vi "EventDisplayWindow.vi"(8 "error in (no error)":errorcluster, 11 "Path to detector WRL file":path) -> (0 "error out":errorcluster)   [LabVIEW 2016]
uses:
  Typedefs/Coincidence.ctl
panel:
  in  "Events/sec":dbl=1.0
  in  "Firing color":u32(colorbox)=9809083
  in  "Idle color":u32(colorbox)=9809083
  in  "Enable Events":bool=TRUE
  in  "Scale":sgl=0.01
  out "Event display":refnum<vi>(3d-picture)
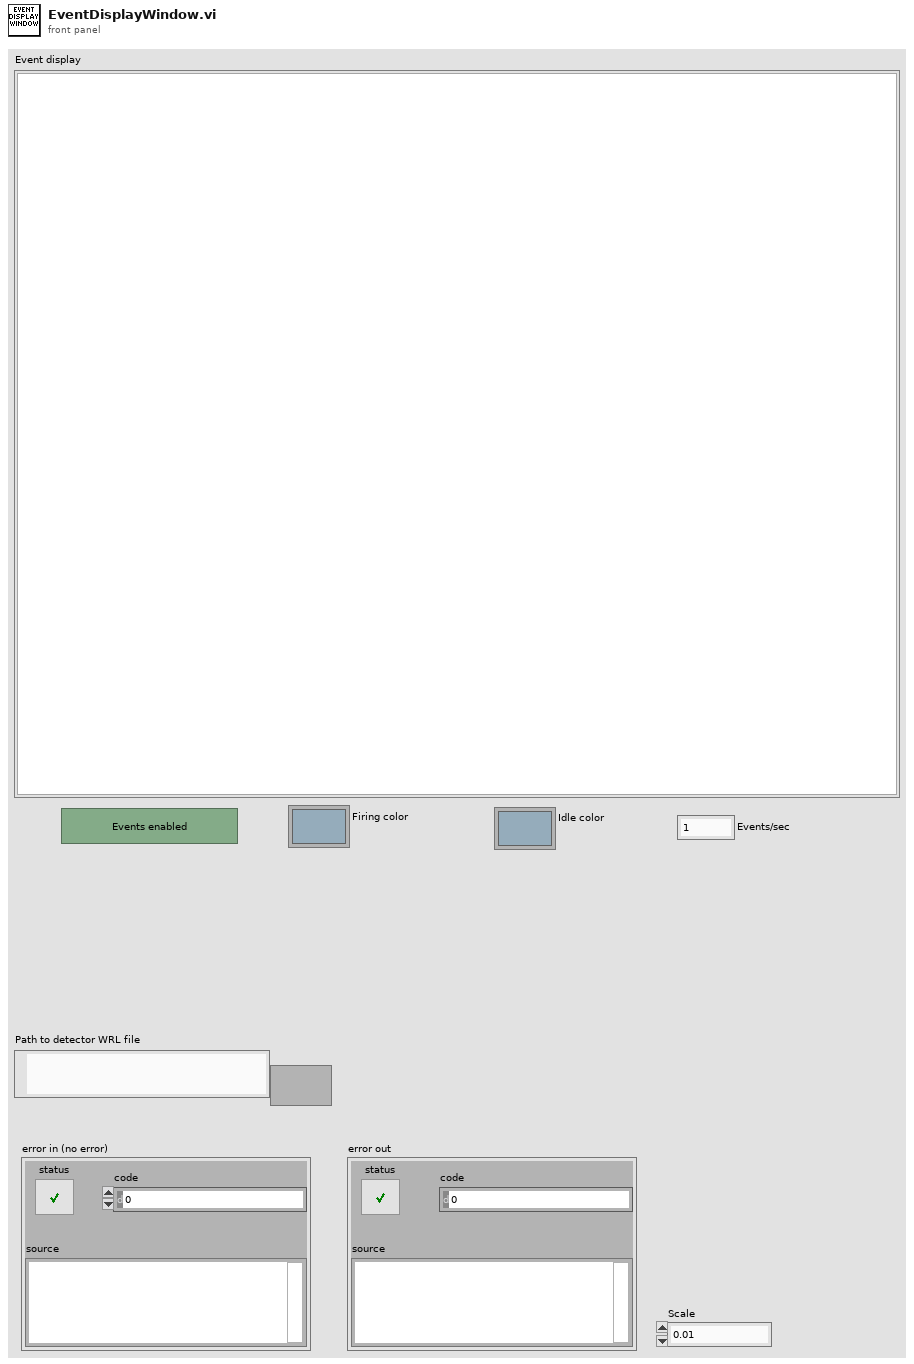
[diagram p1: front panel]
types:
  T1 = typedef "Coincidence.ctl" = cluster{"Primary ID":i8, "Muon hit time":u64, "Secondary ID":i8, "DeltaT":i32}
  T2 = cluster{"Simultaneus muon tracks":cluster{"Top coinc":T1, "Bottom coinc":T1}[]}[]
  T3 = cluster{"Frame color":u32, "Connectors color":u32, "Supports color":u32, "Bolts color":u32, "Scintillators color":u32, "Scintillator alpha":sgl}
  T4 = cluster{"Simultaneus muon tracks":cluster{"Top coinc":T1, "Bottom coinc":T1}[]}
  T5 = typedef "LVRGBAColorTypeDef.ctl" = cluster{"Red":sgl, "Green":sgl, "Blue":sgl, "Alpha":sgl}
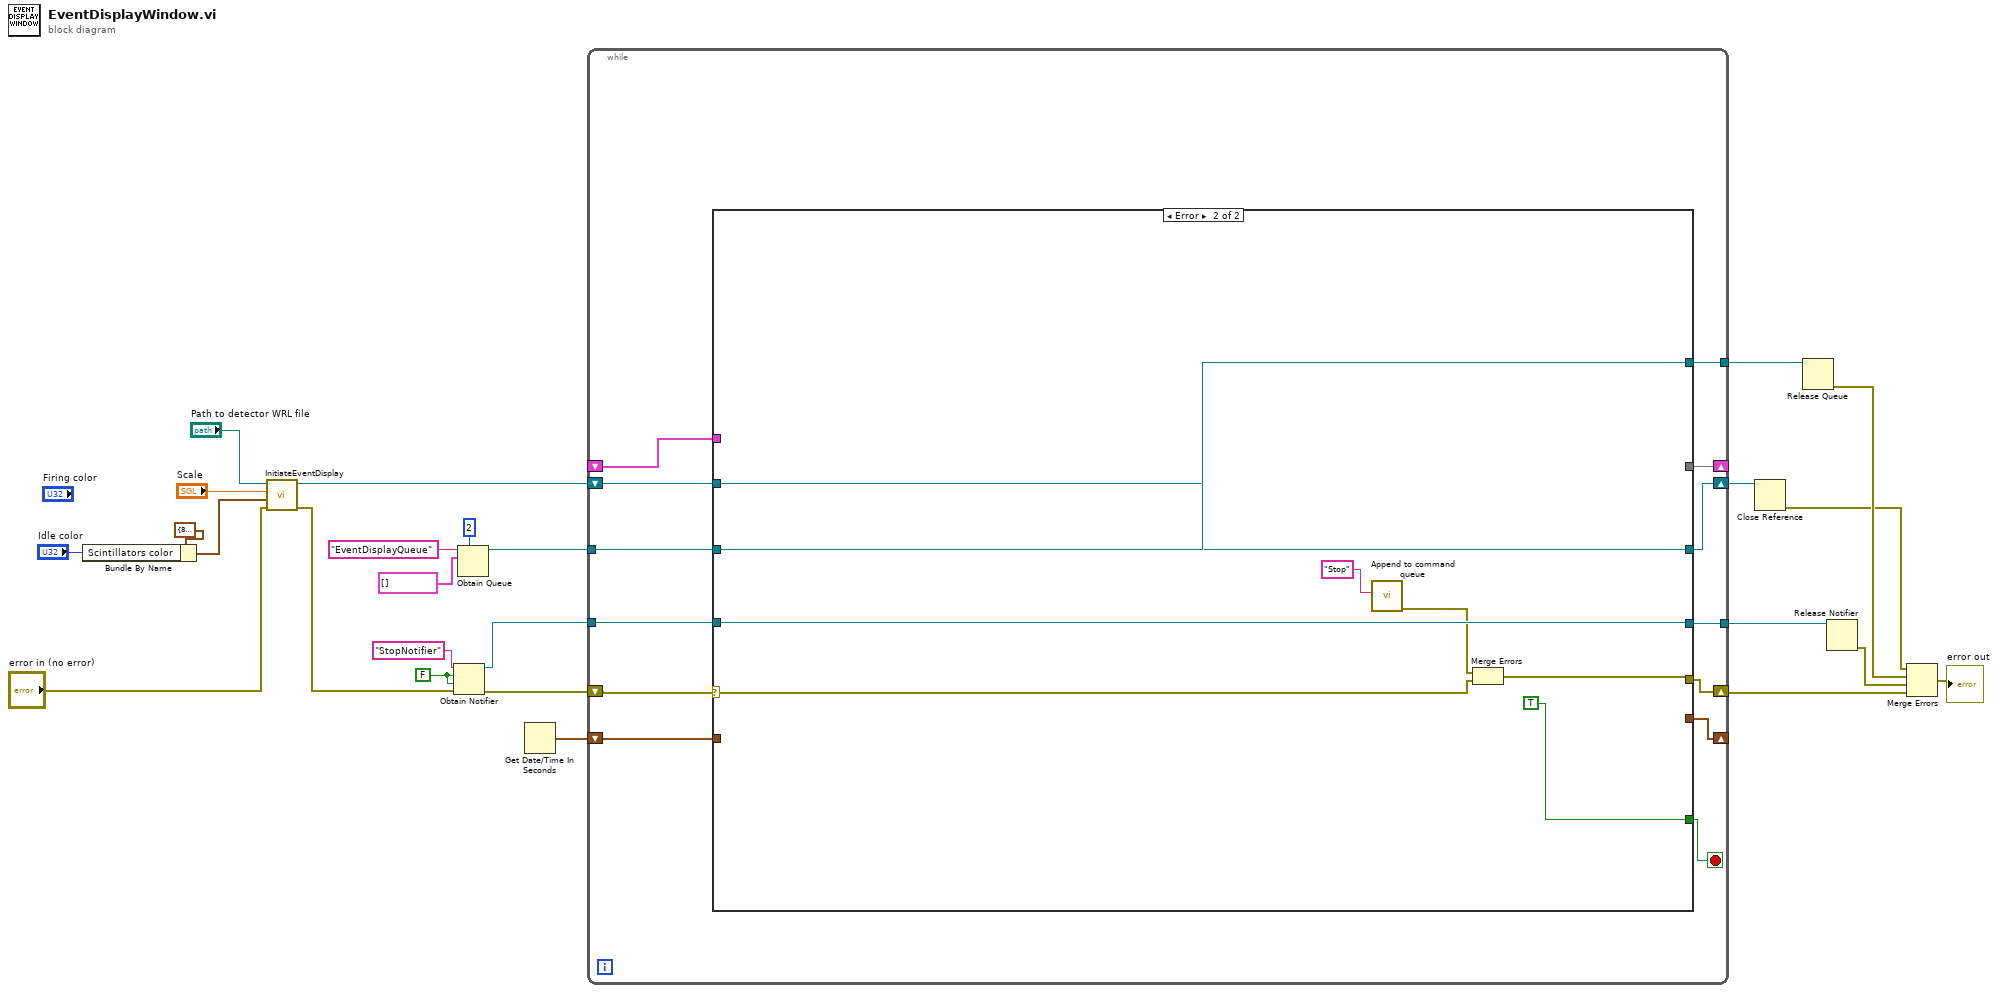
[diagram p0: block diagram]
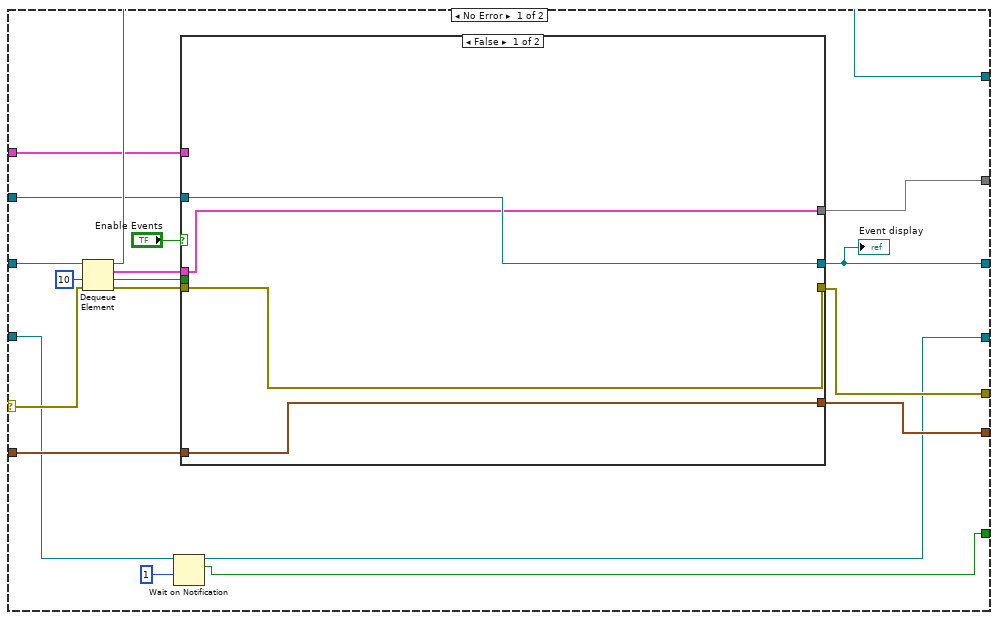
[diagram p2: hidden frame]
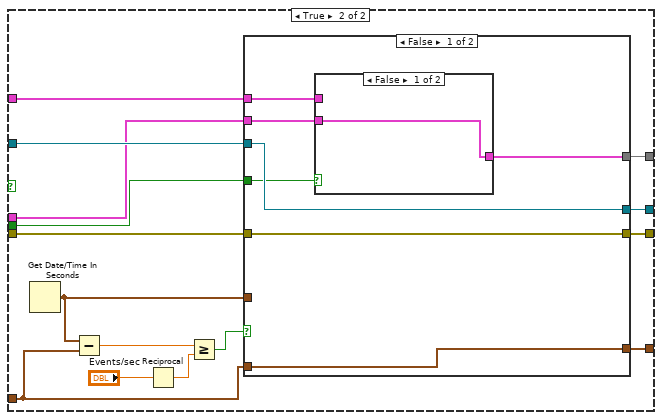
[diagram p3: hidden frame]
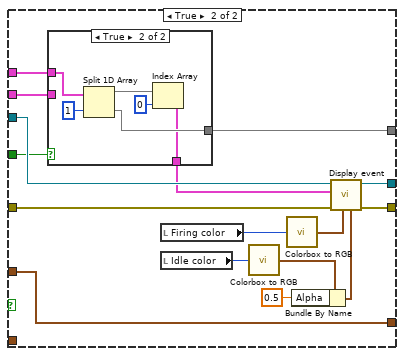
[diagram p5: hidden frame]
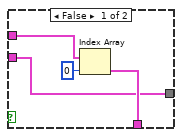
[diagram p6: hidden frame]
diagram:
  w24 = FALSE
  n1 = Bundle By Name(cluster=T3 {"Frame color"=8950380, "Connectors color"=5921370, "Supports color"=10395294, "Bolts color"=13487565, "Scintillators color"=9809083, "Scintillator alpha"=0.5} ("colors"), "Scintillators color"="Idle color") -> (w4:T3)
  n2 = call "InitiateEventDisplay.vi"("error in"="error in (no error)", "colors"=w4, "Scale"="Scale", "Path to detector WRL file"="Path to detector WRL file") -> ("error out"=w9:errorcluster, "Event Display Scene"=w8:refnum<vi>)  [unwired: 4 in]
  n3 = Obtain Notifier(name (unnamed)="StopNotifier", notification data type=w24, create if not found? (T)=w24, error in (no error)=w9) -> (notifier out=w22:refnum<notifier>, error out=w23:errorcluster)  [unwired: 1 out]
  n4 = Obtain Queue(max queue size (-1, unlimited)=2, name (unnamed)="EventDisplayQueue", element data type=T2 []) -> (queue out=w19:refnum<queue>)  [unwired: 2 in, 2 out]
  n5 = Get Date/Time In Seconds() -> (seconds since 1Jan1904=w2:timestamp)
  n6 = while {
    tunnel: w22 -> [w34]
    tunnel: w19 -> [w36]
    shift-right: [w35] -> w14
    shift-left: w23 -> [w38]
    tunnel: [w33] -> w17
    tunnel: [w32] -> w18
    shift-right: [w30] -> w7
    shift-left: w8 -> [w31]
    shift-right: [w28] -> _
    shift-left: w2 -> [w29]
    shift-right: [w26] -> _
    shift-left: _ -> [w27]
    stop <- w37 stop-if-true
    n7 = case shown="Error" w38 {
      selector: w38 -> [w55 w114]
      tunnel: [w44 TRUE] -> w37
      tunnel: w36 -> [w57 w113]
      tunnel: [w54 w116] -> w35
      tunnel: w34 -> [w46 w118]
      tunnel: [w45 w118] -> w33
      tunnel: [w52 w113] -> w32
      tunnel: w31 -> [w51 w112]
      tunnel: [w50 w112] -> w30
      tunnel: w29 -> [w49 _]
      tunnel: [w48 _] -> w28
      tunnel: w27 -> [w39 _]
      tunnel: [w41 _] -> w26
      frame No Error {
        n8 = Dequeue Element(queue=w57, timeout in ms (-1)=10, error in (no error)=w55) -> (queue out=w52:refnum<queue>, element=w42:T2, timed out?=w40:bool, error out=w53:errorcluster)
        n9 = Wait on Notification(notifier=w46, timeout in ms (-1)=1) -> (notifier out=w45:refnum<notifier>, notification=w44:bool)  [unwired: 2 in, 2 out]
        n10 = case shown="False" "Enable Events" {
          tunnel: w53 -> [w60 w76]
          tunnel: [w60 w75] -> w54
          tunnel: w51 -> [w61 w74]
          tunnel: [w61 w73] -> w50
          tunnel: w49 -> [w59 w66]
          tunnel: [w59 w68] -> w48
          tunnel: w42 -> [w58 w65]
          tunnel: [w58 w64] -> w41
          tunnel: w40 -> [_ w63]
          tunnel: w39 -> [_ w62]
          frame False {
          }
          frame True {
            n11 = Get Date/Time In Seconds() -> (seconds since 1Jan1904=w67:timestamp)
            n12 = Subtract(x=w67, y=w66) -> (x-y=w72:dbl)
            n13 = Reciprocal(x="Events/sec") -> (1/x=w70:dbl)
            n14 = Greater Or Equal?(x=w72, y=w70) -> (x >= y?=w69:bool)
            n15 = case shown="False" w69 {
              tunnel: w76 -> [w82 w101]
              tunnel: [w82 w100] -> w75
              tunnel: w74 -> [w83 w99]
              tunnel: [w83 w98] -> w73
              tunnel: [w81 w91] -> w68
              tunnel: w67 -> [_ w91]
              tunnel: w66 -> [w81 _]
              tunnel: w65 -> [w79 w90]
              tunnel: [w77 w89] -> w64
              tunnel: w63 -> [w80 w88]
              tunnel: w62 -> [w78 w86]
              frame False {
                n16 = case shown="False" w80 {
                  tunnel: w79 -> [w84 _]
                  tunnel: w78 -> [_ w85]
                  tunnel: [w84 w85] -> w77
                  frame False {
                  }
                  frame True {
                  }
                }
              }
              frame True {
                n17 = case shown="True" w88 {
                  tunnel: [w103 w110] -> w89
                  tunnel: [w104 w107] -> w87
                  tunnel: w90 -> [w103 _]
                  tunnel: w86 -> [w102 w106]
                  frame False {
                    n18 = Index Array(array=w102, index=0) -> (element=w104:T4)
                  }
                  frame True {
                    n19 = Split 1D Array(array=w106, index=1) -> (first subarray=w109:T2, second subarray=w110:T2)
                    n20 = Index Array(array=w109, index=0) -> (element=w107:T4)
                  }
                }
                n21 = local read "Firing color"() -> (w96:u32)
                n22 = local read "Idle color"() -> (w97:u32)
                n23 = call "Colorbox to RGB.vi"("Color"=w97) -> ("Material"=w94:T5)
                n24 = call "Colorbox to RGB.vi"("Color"=w96) -> ("Material"=w95:T5)
                n25 = Bundle By Name(cluster=w94, "Alpha"=sgl 0.5) -> (w92:T5)
                n26 = call "Display event.vi"("No hit color"=w92, "Hit color"=w95, "error in (no error)"=w101, "Hits to display"=w87, "Event Display in"=w99) -> ("error out"=w100:errorcluster, "Event Display out"=w98:refnum<vi>)  [unwired: 5 in]
              }
            }
          }
        }
        "Event display" <- w50
      }
      frame Error {
        n27 = call "Append to command queue.vi"("Single command"="Stop") -> ("error out"=w115:errorcluster)  [unwired: 10 in]
        n28 = Merge Errors(w115, w114) -> (w116:errorcluster)
      }
    }
  }
  n29 = Close Reference(reference=w7) -> (error out=w3:errorcluster)  [unwired: 1 in]
  n30 = Release Queue(queue=w18) -> (error out=w16:errorcluster)  [unwired: 2 in, 2 out]
  n31 = Release Notifier(notifier=w17) -> (error out=w15:errorcluster)  [unwired: 2 in, 2 out]
  n32 = Merge Errors(w3, w16, w15, w14) -> (→"error out":errorcluster)
